vi "AMC Dispatcher.vi"() -> ()   [LabVIEW 2017]
uses:
  Tools/Keyed Array/Tools_KeyedArray KeyedArray.ctl
  subVIs/TypeDefs/amc_UDP Port Functions.ctl
  subVIs/amc_Globals.vi
panel:
  out "Dispatcher Error":errorcluster
  out "Sender Process":string
  out "Sender":string
  in  "Stop":bool
  out "Message XML String":string
  in  "State Variables":T1={"UDP Conn ID"=refnum, "UDP Port"=54321}
  out "Status":string
  # "Receive"
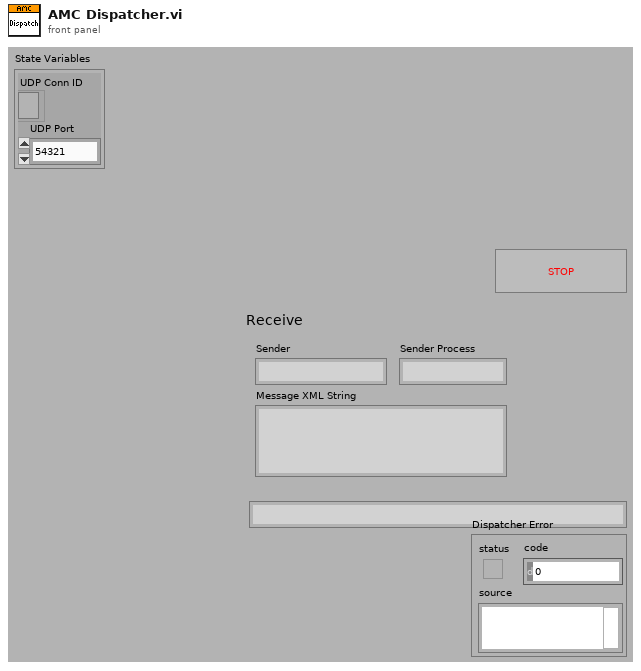
[diagram p1: front panel]
types:
  T1 = cluster{"UDP Conn ID":refnum<k16>, "UDP Port":u16}
  T2 = typedef "amc_Message Queue.ctl" = refnum<queue>
  T3 = typedef "amc_UDP Port Functions.ctl" = enum16{"Init", "Get", "Close"}
  T4 = typedef "Tools_KeyedArray KeyedArray.ctl" = cluster{"keys":string[], "values":string[]}
  T5 = typedef "amc_Message.ctl" = cluster{"Name":string, "Value":string, "Attributes":T4, "Receiver Host":string, "Receiver Process":string, "Source Host":string, "Source Process":string, "Priority Message":bool, "Acknowledge Message":bool}
  T6 = typedef "amc_QueueRegistryProperties.ctl" = cluster{"Name":string}
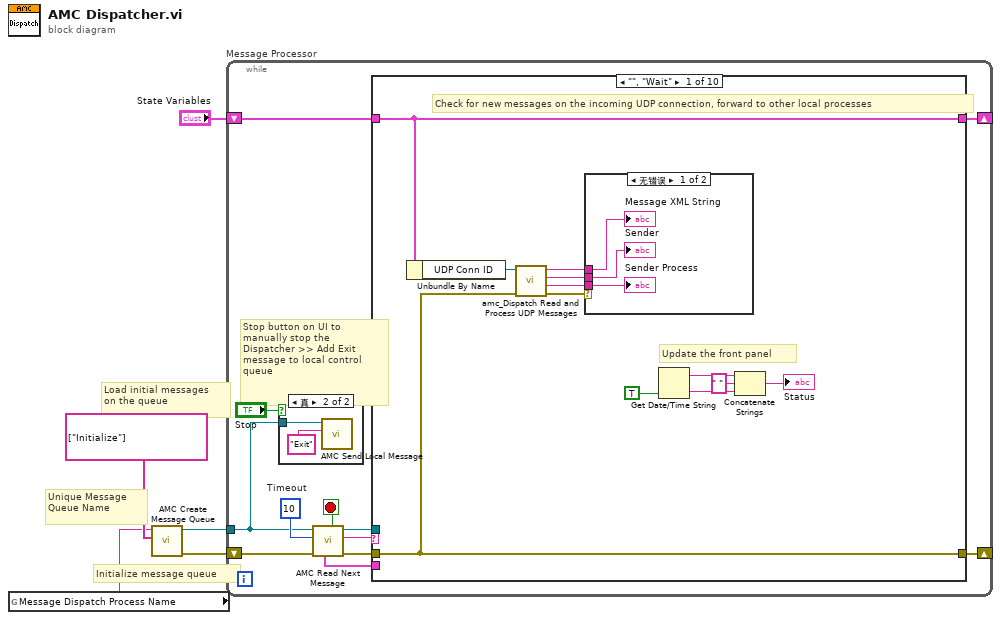
[diagram p0: block diagram]
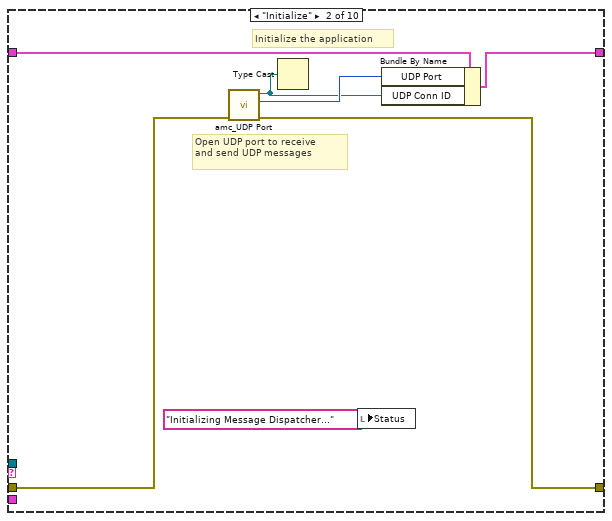
[diagram p4: hidden frame]
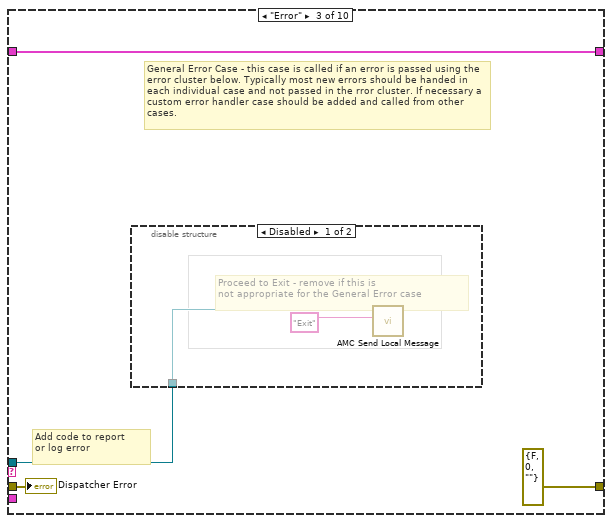
[diagram p5: hidden frame]
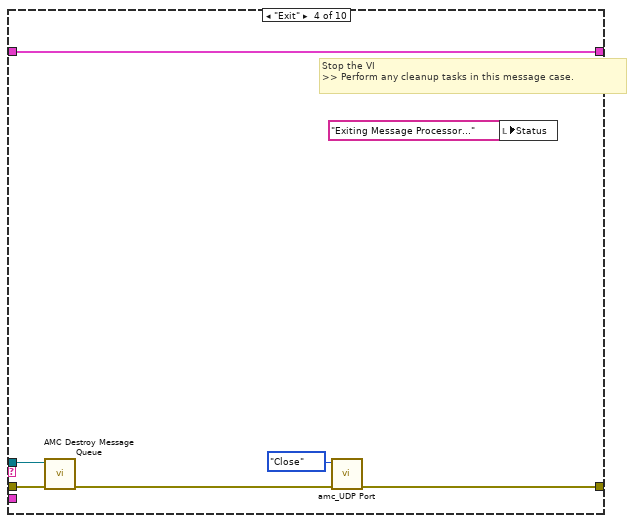
[diagram p7: hidden frame]
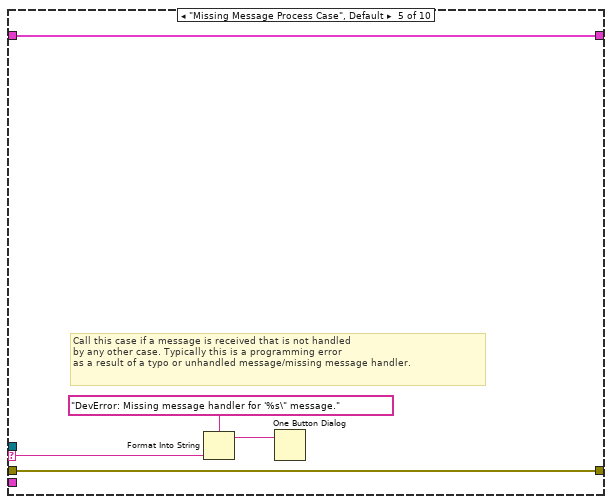
[diagram p8: hidden frame]
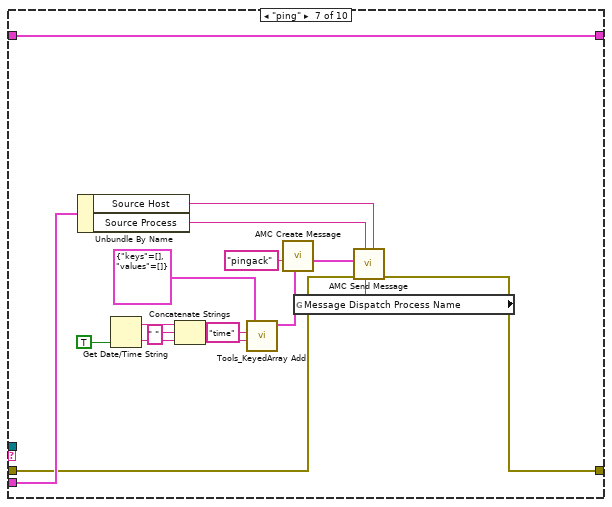
[diagram p10: hidden frame]
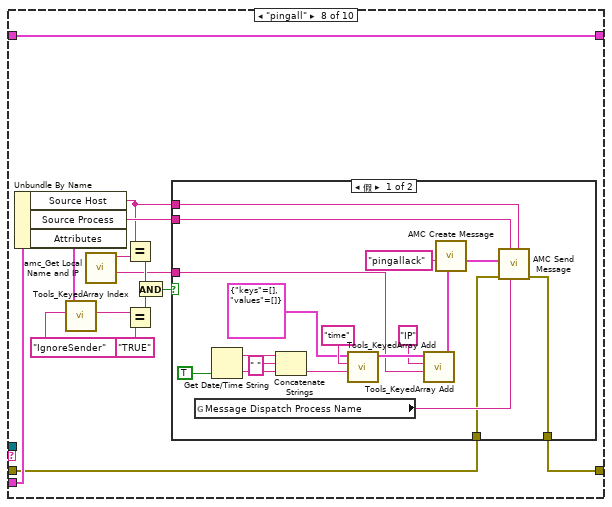
[diagram p11: hidden frame]
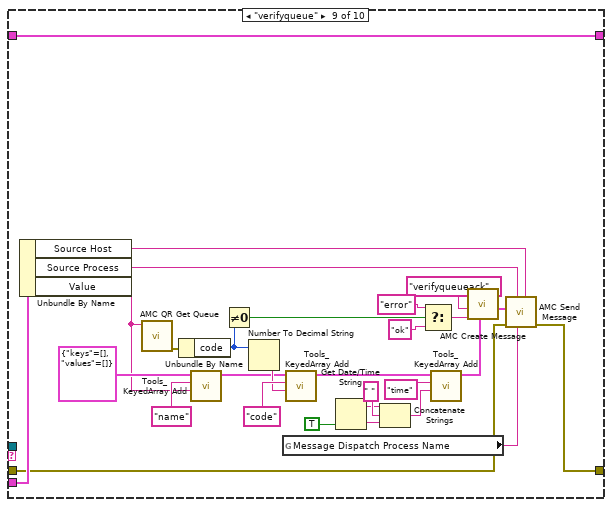
[diagram p13: hidden frame]
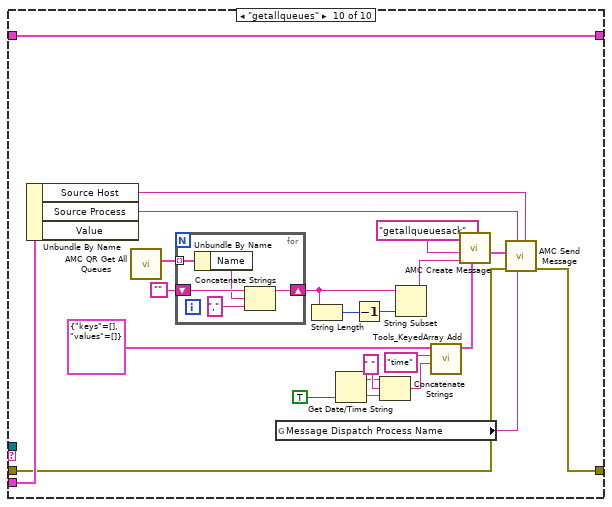
[diagram p14: hidden frame]
diagram:
  # "Initialize message queue"
  # "Unique Message\nQueue Name"
  # "Load initial messages\non the queue"
  n1 = global read "amc_Globals.vi" "Message Dispatch Process Name"() -> (w1:string)
  n2 = call "AMC Create Message Queue.vi"("Initial Message Names"=string[] ["Initialize"], "Message Queue Name"=w1) -> ("error out"=w3:errorcluster, "Message Queue out"=w5:T2)  [unwired: 3 in, 5 out]
  n3 = while "Message Processor" {
    shift-left: w3 -> [w13]
    shift-right: [w14] -> _
    tunnel: w5 -> [w8]
    shift-left: "State Variables" -> [w17]
    shift-right: [w7] -> _
    stop <- w10 stop-if-true
    w12 = 10  # Timeout
    # "Stop button on UI to\nmanually stop the\nDispatcher >> Add Exit\nmessage to local control\nqueue"
    n4 = case shown="真" "Stop" {
      tunnel: w8 -> [_ w18]
      frame False {
      }
      frame True {
        n5 = call "AMC Send Local Message.vi"("Message Name"="Exit", "Message Queue in"=w18) -> ()  [unwired: 4 in, 6 out]
      }
    }
    n6 = call "AMC Read Next Message.vi"("error in (no error)"=w13, "timeout (1ms)"=w12, "Message Queue in"=w8) -> ("error out"=w15:errorcluster, "Message Name"=w11:string, "Message Queue out"=w16:T2, "Exit Process"=w10:bool, "Message"=w6:T5)  [unwired: 1 in, 3 out]
    n7 = case shown="\"\", \"Wait\"" w11 {
      selector: w11 -> [_ _ _ _ w57 _ _ _ _ _]
      tunnel: w17 -> [w26 w40 w45 w52 w59 w61 w78 w93 w141 w164]
      tunnel: w16 -> [_ _ w43 w53 _ _ _ _ _ _]
      tunnel: w15 -> [w20 w37 w42 w54 w58 w60 w63 w80 w114 w143]
      tunnel: [w20 w36 errorcluster {"status"=FALSE, "code"=0, "source"=""} ("error out") w49 w58 w60 w62 w79 w113 w142] -> w14
      tunnel: [w26 w39 w45 w52 w59 w61 w78 w93 w141 w164] -> w7
      tunnel: w6 -> [_ _ _ _ _ _ w75 w92 w139 w162]
      frame "", "Wait" {
        # "Check for new messages on the incoming UDP connection, forward to other local processes"
        # "Update the front panel"
        n8 = Unbundle By Name(w26) -> ("UDP Conn ID"=w22:refnum<k16>)
        n9 = call "amc_Dispatch Read and Process UDP Messages.vi"("error in"=w20, "UDP Conn ID"=w22) -> ("error out"=w21:errorcluster, "Source Process"=w24:string, "Sender Host"=w23:string, "Message XML String"=w25:string)  [unwired: 1 in, 5 out]
        n10 = case shown="无错误" w21 {
          tunnel: w25 -> [w34 _]
          tunnel: w24 -> [w33 _]
          tunnel: w23 -> [w32 _]
          frame No Error {
            "Sender Process" <- w33
            "Sender" <- w32
            "Message XML String" <- w34
          }
          frame Error {
          }
        }
        n11 = Get Date/Time String(want seconds? (F)=TRUE) -> (date string=w31:string, time string=w30:string)  [unwired: 2 out]
        n12 = Concatenate Strings(w31, " " ("string"), w30) -> (→"Status":string)
      }
      frame "Initialize" {
        # "Open UDP port to receive\nand send UDP messages"
        # "Initialize the application"
        n13 = call "amc_UDP Port.vi"("error in (no error)"=w37) -> ("error out"=w36:errorcluster, "UDP Port"=w38:u16, "UDP Port Ref"=w35:refnum<k16>)  [unwired: 2 in, 6 out]
        n14 = Type Cast(x=w35) -> ()  [unwired: 2 out]
        n15 = local write "Status"("Initializing Message Dispatcher..." ("message")) -> ()
        n16 = Bundle By Name(cluster=w40, "UDP Port"=w38, "UDP Conn ID"=w35) -> (w39:T1)
      }
      frame "Error" {
        # "Add code to report\nor log error"
        # "General Error Case - this case is called if an error is passed using the error cluster below. Typically most new errors should be handed in each individual case and not passed in the rror cluster. If necessary a custom error handler case should be added and called from other cases."
        n17 = disable-structure shown="Disabled" {
          disable-tunnel: w43 -> [w47 _]
          frame Disabled {
            # "Proceed to Exit - remove if this is\nnot appropriate for the General Error case"
            n18 = call "AMC Send Local Message.vi"("Message Name"="Exit", "Message Queue in"=w47) -> ()  [unwired: 4 in, 6 out]
          }
          frame Enabled {
          }
        }
        "Dispatcher Error" <- w42
      }
      frame "Exit" {
        # "Stop the VI\n>> Perform any cleanup tasks in this message case."
        n19 = call "AMC Destroy Message Queue.vi"("error in (no error)"=w54, "Message Queue in"=w53) -> ("error out"=w48:errorcluster)  [unwired: 9 out]
        n20 = call "amc_UDP Port.vi"("error in (no error)"=w48, "UDP Port Functions"=amc_UDP_Port_Functions."Close") -> ("error out"=w49:errorcluster)  [unwired: 9 out]
        n21 = local write "Status"("Exiting Message Processor..." ("button name (\"OK\")")) -> ()
      }
      frame "Missing Message Process Case", Default {
        # "Call this case if a message is received that is not handled \nby any other case. Typically this is a programming error\nas a result of a typo or unhandled message/missing message handler."
        n22 = Format Into String(format string="DevError: Missing message handler for '%s\" message." ("message"), w57) -> (resulting string=w55:string)  [unwired: 2 in, 1 out]
        n23 = One Button Dialog(message=w55) -> ()  [unwired: 2 out]
      }
      frame "**** Message Dispatcher Service Functions ****" {
      }
      frame "ping" {
        n24 = Unbundle By Name(w75) -> ("Source Host"=w73:string, "Source Process"=w74:string)
        n25 = Get Date/Time String(want seconds? (F)=TRUE) -> (date string=w72:string, time string=w71:string)  [unwired: 2 out]
        n26 = Concatenate Strings(w72, " ", w71) -> (w69:string)
        n27 = call "Tools_KeyedArray Add.vi"("value"=w69, "key"="time", "array in"=T4 {"keys"=[], "values"=[]}) -> ("array out"=w67:T4)  [unwired: 1 in, 3 out]
        n28 = call "AMC Create Message.vi"("Attributes"=w67, "Name"="pingack") -> ("Message"=w77:T5)  [unwired: 1 in, 8 out]
        n29 = global read "amc_Globals.vi" "Message Dispatch Process Name"() -> (w64:string)
        n30 = call "AMC Send Message.vi"("Receiver Host"=w73, "Source Process"=w64, "Receiver Process"=w74, "error in (no error)"=w63, "Message"=w77) -> ("error out"=w62:errorcluster)  [unwired: 3 in, 3 out]
      }
      frame "pingall" {
        n31 = Unbundle By Name(w92) -> ("Source Host"=w81:string, "Source Process"=w87:string, "Attributes"=w91:T4)
        n32 = call "Tools_KeyedArray Index.vi"("key"="IgnoreSender", "array in"=w91) -> ("value"=w89:string)  [unwired: 2 in, 3 out]
        n33 = call "amc_Get Local Name and IP.vi"() -> ("IP Address"=w82:string, "Name"=w83:string)  [unwired: 1 in, 9 out]
        n34 = Equal?(x=w81, y=w83) -> (x = y?=w85:bool)
        n35 = Equal?(x=w89, y="TRUE" ("x")) -> (x = y?=w86:bool)
        n36 = And(x=w85, y=w86) -> (x .and. y?=w84:bool)
        n37 = case shown="假" w84 {
          tunnel: w81 -> [w111 _]
          tunnel: w87 -> [w110 _]
          tunnel: w82 -> [w97 _]
          tunnel: w80 -> [w95 w112]
          tunnel: [w94 w112] -> w79
          frame False {
            n38 = global read "amc_Globals.vi" "Message Dispatch Process Name"() -> (w96:string)
            n39 = Get Date/Time String(want seconds? (F)=TRUE) -> (date string=w107:string, time string=w106:string)  [unwired: 2 out]
            n40 = Concatenate Strings(w107, " ", w106) -> (w104:string)
            n41 = call "Tools_KeyedArray Add.vi"("value"=w104, "key"="time", "array in"=T4 {"keys"=[], "values"=[]}) -> ("array out"=w100:T4)  [unwired: 1 in, 3 out]
            n42 = call "Tools_KeyedArray Add.vi"("value"=w97, "key"="IP", "array in"=w100) -> ("array out"=w99:T4)  [unwired: 1 in, 3 out]
            n43 = call "AMC Create Message.vi"("Attributes"=w99, "Name"="pingallack") -> ("Message"=w109:T5)  [unwired: 1 in, 8 out]
            n44 = call "AMC Send Message.vi"("Receiver Host"=w111, "Source Process"=w96, "Receiver Process"=w110, "error in (no error)"=w95, "Message"=w109) -> ("error out"=w94:errorcluster)  [unwired: 3 in, 3 out]
          }
          frame True {
            # "Do not respond if the PingAll request was sent by this system"
          }
        }
      }
      frame "verifyqueue" {
        n45 = Unbundle By Name(w139) -> ("Source Host"=w137:string, "Source Process"=w138:string, "Value"=w117:string)
        n46 = call "AMC QR Get Queue .vi"("Name"=w117) -> ("error out"=w116:errorcluster)  [unwired: 1 in, 9 out]
        n47 = Unbundle By Name(w116) -> ("code"=w130:i32)
        n48 = call "Tools_KeyedArray Add.vi"("value"=w117, "key"="name", "array in"=T4 {"keys"=[], "values"=[]}) -> ("array out"=w132:T4)  [unwired: 1 in, 3 out]
        n49 = Not Equal To 0?(x=w130) -> (x != 0?=w129:bool)
        n50 = Number To Decimal String(number=w130) -> (decimal integer string=w134:string)  [unwired: 1 out]
        n51 = global read "amc_Globals.vi" "Message Dispatch Process Name"() -> (w115:string)
        n52 = call "Tools_KeyedArray Add.vi"("value"=w134, "key"="code", "array in"=w132) -> ("array out"=w119:T4)  [unwired: 1 in, 3 out]
        n53 = Get Date/Time String(want seconds? (F)=TRUE) -> (date string=w123:string, time string=w122:string)  [unwired: 2 out]
        n54 = Concatenate Strings(w123, " ", w122) -> (w121:string)
        n55 = Select(t="error", s=w129, f="ok") -> (s? t:f=w128:string)
        n56 = call "Tools_KeyedArray Add.vi"("value"=w121, "key"="time", "array in"=w119) -> ("array out"=w118:T4)  [unwired: 1 in, 3 out]
        n57 = call "AMC Create Message.vi"("Attributes"=w118, "Value"=w128, "Name"="verifyqueueack") -> ("Message"=w140:T5)  [unwired: 8 out]
        n58 = call "AMC Send Message.vi"("Receiver Host"=w137, "Source Process"=w115, "Receiver Process"=w138, "error in (no error)"=w114, "Message"=w140) -> ("error out"=w113:errorcluster)  [unwired: 3 in, 3 out]
      }
      frame "getallqueues" {
        n59 = Unbundle By Name(w162) -> ("Source Host"=w160:string, "Source Process"=w161:string)  [unwired: 1 out]
        n60 = call "AMC QR Get All Queues.vi"() -> ("All Properties"=w151:T6[])  [unwired: 1 in, 10 out]
        n61 = for {
          shift-right: [w169] -> w147
          shift-left: "" -> [w168]
          tunnel: w151 -> [w167] mode=indexing
          n62 = Unbundle By Name(w167) -> ("Name"=w166:string)
          n63 = Concatenate Strings(w168, w166, "," ("string")) -> (w169:string)
        }
        n64 = global read "amc_Globals.vi" "Message Dispatch Process Name"() -> (w144:string)
        n65 = String Length(string=w147) -> (length=w149:i32)
        n66 = Get Date/Time String(want seconds? (F)=TRUE) -> (date string=w156:string, time string=w155:string)  [unwired: 2 out]
        n67 = Decrement(x=w149) -> (x-1=w148:i32)
        n68 = Concatenate Strings(w156, " ", w155) -> (w154:string)
        n69 = String Subset(string=w147, length (rest)=w148) -> (substring=w146:string)  [unwired: 1 out]
        n70 = call "Tools_KeyedArray Add.vi"("value"=w154, "key"="time", "array in"=T4 {"keys"=[], "values"=[]}) -> ("array out"=w152:T4)  [unwired: 1 in, 3 out]
        n71 = call "AMC Create Message.vi"("Attributes"=w152, "Value"=w146, "Name"="getallqueuesack") -> ("Message"=w163:T5)  [unwired: 8 out]
        n72 = call "AMC Send Message.vi"("Receiver Host"=w160, "Source Process"=w144, "Receiver Process"=w161, "error in (no error)"=w143, "Message"=w163) -> ("error out"=w142:errorcluster)  [unwired: 3 in, 3 out]
      }
    }
  }
